vi "Drive_Execute.vi"   [LabVIEW 2019]
uses:
  Globals/Drive_Globals.vi
types:
  T1 = typedef "Drive_Cluster.ctl" = cluster{"Control_State":T2, "Vertical_Throttle":dbl, "Lateral_Throttle":dbl, "Rotational_Throttle":dbl}
  T2 = typedef "Drive_States.ctl" = enum16{"Manual_Swerve_Math", ""}
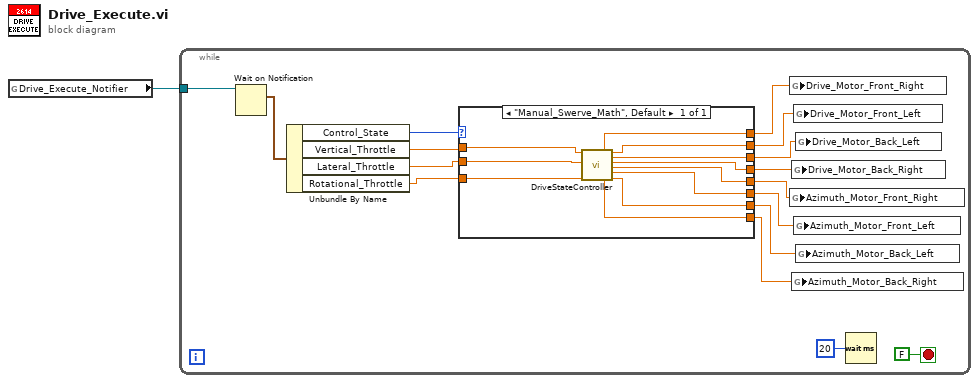
[diagram p0: block diagram]
diagram:
  n1 = global read "Drive_Globals.vi" "Drive_Execute_Notifier"() -> (w1:refnum<notifier>)
  n2 = while {
    tunnel: w1 -> [w15]
    stop <- FALSE stop-if-true
    n3 = Wait on Notification(notifier=w15) -> (notification=w14:T1)  [unwired: 3 in, 3 out]
    n4 = Unbundle By Name(w14) -> ("Control_State"=w13:T2, "Vertical_Throttle"=w4:dbl, "Lateral_Throttle"=w3:dbl, "Rotational_Throttle"=w2:dbl)
    n5 = case shown="\"Manual_Swerve_Math\", Default" w13 {
      tunnel: [w28] -> w12
      tunnel: [w27] -> w11
      tunnel: [w26] -> w10
      tunnel: [w25] -> w9
      tunnel: [w24] -> w8
      tunnel: [w23] -> w7
      tunnel: [w22] -> w6
      tunnel: [w21] -> w5
      tunnel: w4 -> [w20]
      tunnel: w3 -> [w19]
      tunnel: w2 -> [w18]
      frame "Manual_Swerve_Math", Default {
        n6 = call "DriveStateController.vi"("Vertical_Throttle"=w20, "Lateral_Throttle"=w19, "Rotational_Throttle"=w18) -> ("Drive_Motor_Front_Right"=w28:dbl, "Azimuth_Motor_Back_Right"=w21:dbl, "Drive_Motor_Front_Left"=w27:dbl, "Drive_Motor_Back_Left"=w26:dbl, "Drive_Motor_Back_Right"=w25:dbl, "Azimuth_Motor_Front_Right"=w24:dbl, "Azimuth_Motor_Front_Left"=w23:dbl, "Azimuth_Motor_Back_Left"=w22:dbl)  [unwired: 9 in]
      }
    }
    n7 = global write "Drive_Globals.vi" "Drive_Motor_Front_Right"(w12) -> ()
    n8 = global write "Drive_Globals.vi" "Azimuth_Motor_Front_Right"(w8) -> ()
    n9 = global write "Drive_Globals.vi" "Drive_Motor_Back_Right"(w9) -> ()
    n10 = global write "Drive_Globals.vi" "Azimuth_Motor_Back_Right"(w5) -> ()
    n11 = global write "Drive_Globals.vi" "Drive_Motor_Front_Left"(w11) -> ()
    n12 = global write "Drive_Globals.vi" "Azimuth_Motor_Front_Left"(w7) -> ()
    n13 = global write "Drive_Globals.vi" "Drive_Motor_Back_Left"(w10) -> ()
    n14 = global write "Drive_Globals.vi" "Azimuth_Motor_Back_Left"(w6) -> ()
    n15 = Wait (ms)(milliseconds to wait=u32 20) -> ()  [unwired: 1 out]
  }
